vi "XPath Example.vi"(8 "error in (no error)":errorcluster) -> (0 "error out":errorcluster)   [LabVIEW 2016, in "SLL File IO.lvlib"]
uses:
  SLL File IO.lvlib
  _SubVIs/Initialize XML from String.vi
  _SubVIs/Get XPath Text.vi
panel:
  out "Found?":bool
  out "Node Text":string
  in  "XPath Expression":string
  in  "XML String":string
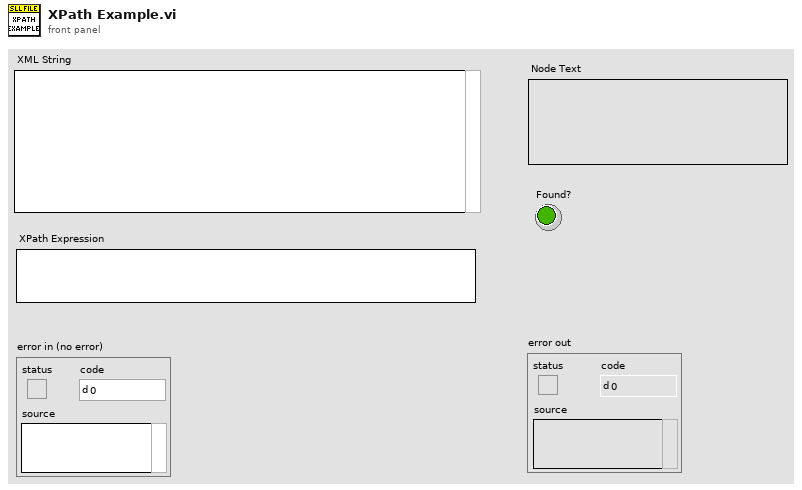
[diagram p1: front panel]
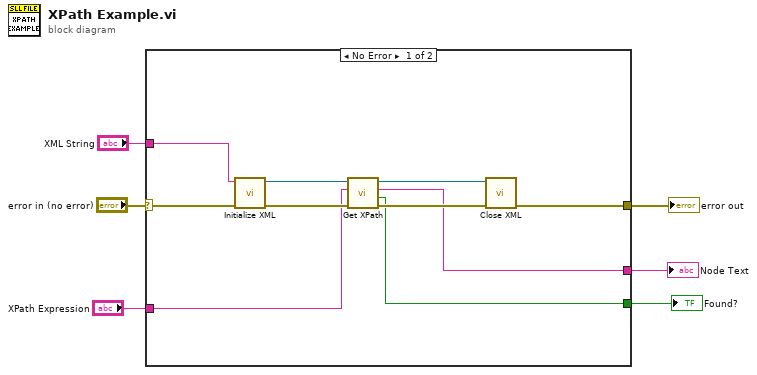
[diagram p0: block diagram]
diagram:
  n1 = case shown="No Error" "error in (no error)" {
    selector: "error in (no error)" -> [w16 w17]
    tunnel: [w10 w17] -> w5
    tunnel: "XML String" -> [w14 _]
    tunnel: "XPath Expression" -> [w11 _]
    tunnel: [w8 _] -> w2
    tunnel: [w7 _] -> w1
    frame No Error {
      n2 = call-poly "Initialize XML.vi"("error in (no error)"=w16, "XML String"=w14) -> ("error out"=w15:errorcluster, "DOM document out"=w12:refnum<k20>)  [unwired: 8 in]
      n3 = call-poly "Get XPath.vi"("error in (no error)"=w15, "XPath Expression"=w11, "DOM document in"=w12) -> ("error out"=w13:errorcluster, "Found?"=w7:bool, "Node Text"=w8:string, "DOM document out"=w9:refnum<k20>)  [unwired: 5 in]
      n4 = call "Close XML.vi"("error in (no error)"=w13, "DOM document in"=w9) -> ("error out"=w10:errorcluster)  [unwired: 9 in]
    }
    frame Error {
    }
  }
  "error out" <- w5
  "Node Text" <- w2
  "Found?" <- w1
